vi "tkrsa6100 Revision Query.vi"(8 "error in (no error)":errorcluster, 11 "VISA Resource Name":refnum<visa-resource-name>) -> (0 "error out":errorcluster {"code" format="%#.0f"}, 1 "Instrument SN":string, 2 "Instrument Driver Version":string, 3 "dup VISA Resource Name":refnum<visa-resource-name>, 4 "Instrument FW Version":string, 5 "Instrument Type":string)   [LabVIEW 2020, in "Library Instrument & Equipement.lvlib" / "Library Spectrum Analyser.lvlib"]
doc: "This VI queries the instrument for its type, s/n, and fw version. It also returns the instrument driver version information.\n\nFirst error in (no error) is checked for any pending error by tkrsa6100 Write/Read wError Query.vi for any pending errors .\n\nIf error in status is ERROR:\n\nerror in (no error) and VISA Resource Name are passed straight through to error out and dup VISA Resource Name. The VI does not execute. No commands are processed.\n\nIf error in status is NO ERROR:\n\nThe *IDN? query is sent by tkrsa6100 Write/Read wError Query.vi to the instrument. The instrument response string is then parsed to remove the instrument type, s/n, and firmware version information using the Match Pattern function. String indicators Instrument Type, Instrument SN, Instrument FW Version, and Instrument Driver Version are updated with the appropriate information parsed from the entire response string.\n\ndup VISA Resource Name, error out, string indicators Instrument Type, Instrument SN, Instrument FW Version, and Instrument Driver Version are returned to the calling function. \n\nModification History:\n\nRSA6100 Inst Driver Ver. 2.0\nBus Type: GPIB\nRSA6106A, RSA6114A Real-Time Spectrum Analyzer\nCreated By: Tektronix, Inc.\nRelease Date: 2/6/07\nOriginally developed for LabVIEW Ver. 7\nTested with instrument firmware version 1.1.62\nUnsupported command groups: None\n\nRSA6100 Inst Driver Ver. 3.0\nBus Type: GPIB\nRSA6106A, RSA6114A Real-Time Spectrum Analyzer\nCreated By: Tektronix, Inc.\nRelease Date: 12/17/07\nOriginally developed for LabVIEW Ver. 7\nTested with instrument firmware version 1.2.90\nUnsupported command groups: None\n\nRSA6100 Inst Driver Ver. 4.0\nBus Type: GPIB\nRSA6106A, RSA6114A Real-Time Spectrum Analyzer\nCreated By: Tektronix, Inc.\nRelease Date: 3/17/08\nOriginally developed for LabVIEW Ver. 7\nTested with instrument firmware version 1.3.64\nUnsupported command groups: None"
uses:
  Library Spectrum Analyser.lvlib
panel:
  # "RSA6100 Revision Query Driver"
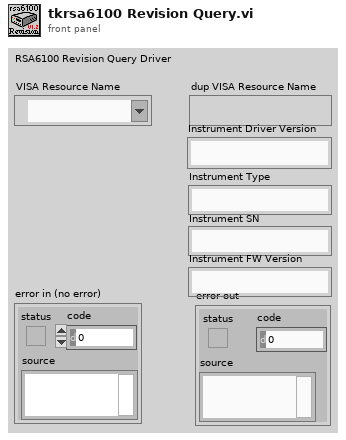
[diagram p1: front panel]
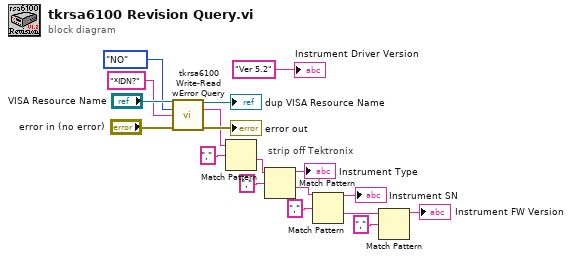
[diagram p0: block diagram]
diagram:
  # "strip off Tektronix"
  n1 = call "tkrsa6100 Write-Read wError Query.vi"("VISA Resource Name"="VISA Resource Name", "Error Query(YES)"=enum16{"NO", "YES"}."NO", "Command (Empty String)"="*IDN?" ("Command"), "error in (no error)"="error in (no error)") -> ("dup VISA Resource Name"=→"dup VISA Resource Name":refnum<visa-resource-name>, "Response"=w4:string, "error out"=→"error out":errorcluster)  [unwired: 3 in, 6 out]
  n2 = Match Pattern(string=w4, regular expression=",") -> (after substring=w12:string)  [unwired: 4 out]
  n3 = Match Pattern(string=w12, regular expression=",") -> (before substring=→"Instrument Type":string, after substring=w6:string)  [unwired: 3 out]
  n4 = Match Pattern(string=w6, regular expression=",") -> (before substring=→"Instrument SN":string, after substring=w5:string)  [unwired: 3 out]
  n5 = Match Pattern(string=w5, regular expression=",") -> (before substring=→"Instrument FW Version":string)  [unwired: 4 out]
  "Instrument Driver Version" <- "Ver 5.2" ("Instrument Driver Version")
